vi "Destroy.vi"(0 "reference in":refnum<class "G#BaseAggregator.lvclass">, 5 "error in (no error)":errorcluster) -> (14 "reference out":refnum<class "G#BaseAggregator.lvclass">, 19 "error out":errorcluster)   [LabVIEW 2020, in "G#BaseAggregator.lvclass"]
doc: "Destructor."
uses:
  G#BaseAggregator.lvclass
  <vilib>/addons/_AddQ/G#Object/G#Object.lvclass
  G#BaseClass1_class/G#BaseClass1.lvclass
  G#BaseClass2_class/G#BaseClass2.lvclass
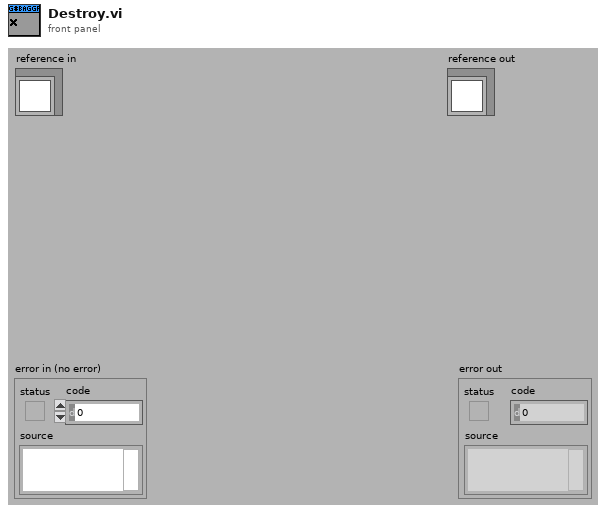
[diagram p1: front panel]
types:
  T1 = typedef "G#BaseAggregator.lvclass/ObjectAttributes.ctl" = cluster{"Numeric":dbl, "G#BaseClass1.lvclass":refnum<class "G#BaseClass1.lvclass">, "G#BaseClass2.lvclass":refnum<class "G#BaseClass2.lvclass">}
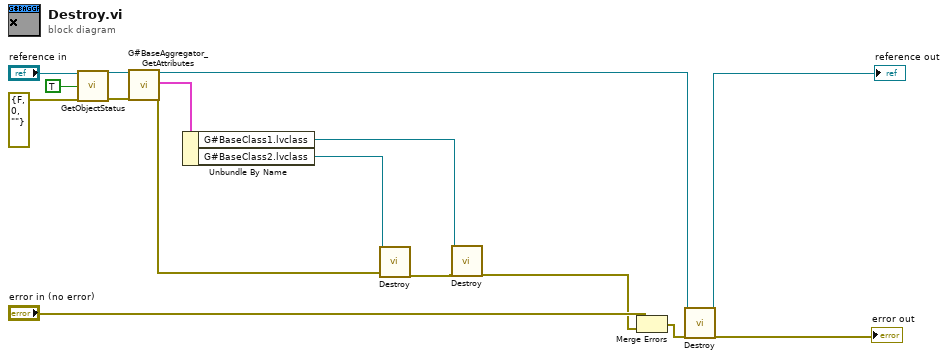
[diagram p0: block diagram]
diagram:
  n1 = call-dynamic "GetObjectStatus.vi"("reference in"="reference in", "simple info (F)"=TRUE ("simple info"), "error in (no error)"=errorcluster {"status"=FALSE, "code"=0, "source"=""}) -> ("reference out"=w10:refnum<class "G#BaseAggregator.lvclass">, "error out"=w11:errorcluster)  [unwired: 5 in, 10 out]
  n2 = call "G#BaseAggregator_GetAttributes.vi"("reference in"=w10, "error in (no error)"=w11) -> ("reference out"=w9:refnum<class "G#BaseAggregator.lvclass">, "attributes"=w8:T1, "error out"=w5:errorcluster)  [unwired: 14 in, 1 out]
  n3 = Unbundle By Name(w8) -> ("G#BaseClass1.lvclass"=w1:refnum<class "G#BaseClass1.lvclass">, "G#BaseClass2.lvclass"=w4:refnum<class "G#BaseClass2.lvclass">)
  n4 = call-dynamic "Destroy.vi"("reference in"=w4, "error in (no error)"=w5) -> ("error out"=w3:errorcluster)  [unwired: 16 in, 1 out]
  n5 = call-dynamic "Destroy.vi"("reference in"=w1, "error in (no error)"=w3) -> ("error out"=w2:errorcluster)  [unwired: 16 in, 1 out]
  n6 = Merge Errors("error in (no error)", w2) -> (w15:errorcluster)
  n7 = call-parent "Destroy.vi"("reference in"=w9, "error in (no error)"=w15) -> ("reference out"=→"reference out":refnum<class "G#BaseAggregator.lvclass">, "error out"=→"error out":errorcluster)  [unwired: 16 in]
